vi "Combined Sim SubVI for 6.0.vi"(2 "Pressure Controls":T1, 3 "Line Flowrate Control":T1, 4 "Temperatures Control":T1) -> (0 "Flow Data":T3(array[cluster]), 1 "Rig Temperatures":T2)   [LabVIEW 2018]
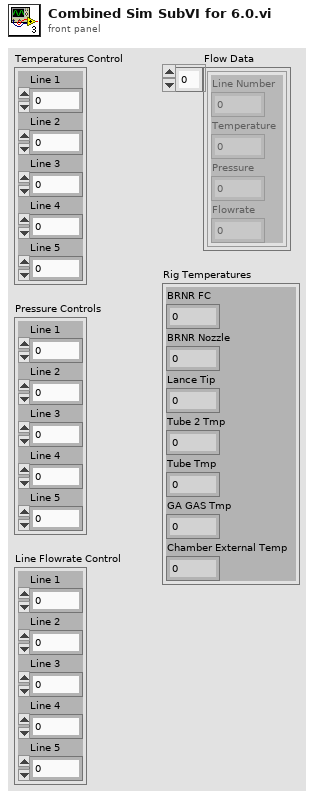
[diagram p1: front panel]
types:
  T1 = cluster{"Line 1":dbl, "Line 2":dbl, "Line 3":dbl, "Line 4":dbl, "Line 5":dbl}
  T2 = cluster{"BRNR FC":dbl, "BRNR Nozzle":dbl, "Lance Tip":dbl, "Tube 2 Tmp":dbl, "Tube Tmp":dbl, "GA GAS Tmp":dbl, "Chamber External Temp":dbl}
  T3 = cluster{"Line Number":dbl, "Temperature":dbl, "Pressure":dbl, "Flowrate":dbl}[]
  T4 = cluster{"Line Number":dbl, "Temperature":dbl, "Pressure":dbl, "Flowrate":dbl}
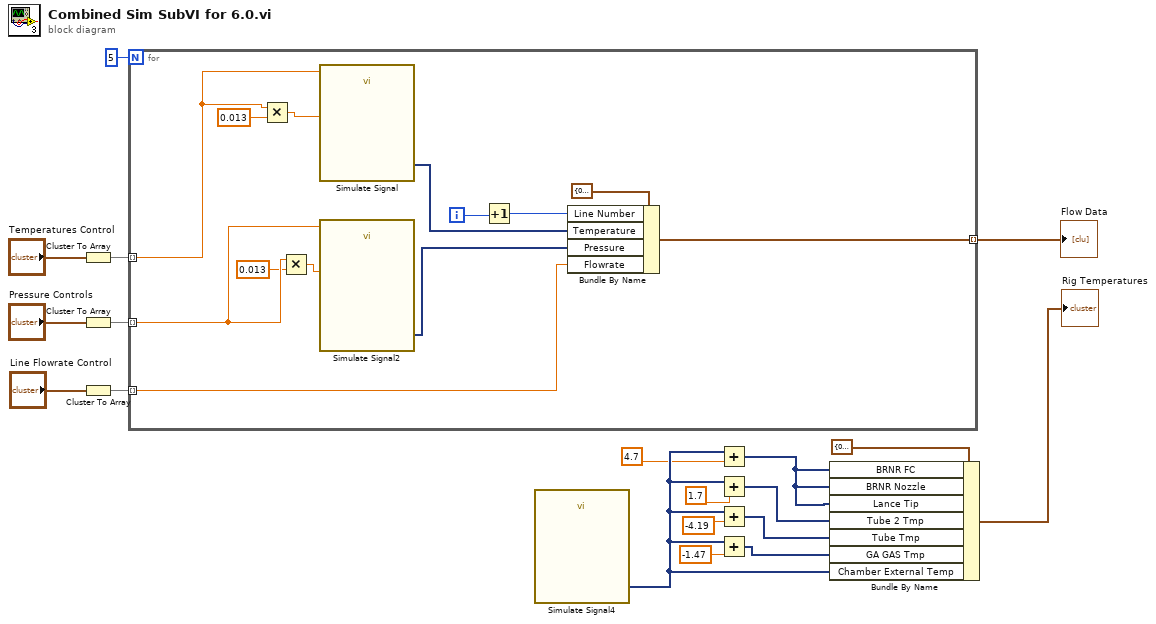
[diagram p0: block diagram]
diagram:
  n1 = Cluster To Array(cluster="Temperatures Control") -> (array=w12:dbl[])
  n2 = Cluster To Array(cluster="Pressure Controls") -> (array=w13:dbl[])
  n3 = Cluster To Array(cluster="Line Flowrate Control") -> (array=w14:dbl[])
  n4 = for {
    N: 5 -> [_]
    tunnel: [w32] -> w19 mode=indexing
    tunnel: w14 -> [w26] mode=indexing
    tunnel: w12 -> [w20] mode=indexing
    tunnel: w13 -> [w25] mode=indexing
    i -> [w30]
    n5 = Multiply(x=w20, y=0.013) -> (x*y=w21:dbl)
    n6 = Multiply(x=w25, y=0.013) -> (x*y=w23:dbl)
    n7 = call "Simulate Signal"("Offset"=w20, "Standard deviation"=w21) -> ("Temperature"=w29:dynamicdata)  [unwired: 12 in, 1 out]
    n8 = call "Simulate Signal2"("Offset"=w25, "Standard deviation"=w23) -> ("Pressure"=w27:dynamicdata)  [unwired: 12 in, 1 out]
    n9 = Increment(x=w30) -> (x+1=w28:i32)
    n10 = Bundle By Name(cluster=T4 {"Line Number"=0.0, "Temperature"=0.0, "Pressure"=0.0, "Flowrate"=0.0}, "Line Number"=w28, "Temperature"=w29, "Pressure"=w27, "Flowrate"=w26) -> (w32:T4)
  }
  "Flow Data" <- w19
  n11 = call "Simulate Signal4"() -> ("Rig Temperatures"=w10:dynamicdata)  [unwired: 14 in, 1 out]
  n12 = Add(x=w10, y=4.7) -> (x+y=w2:dynamicdata)
  n13 = Add(x=w10, y=1.7) -> (x+y=w4:dynamicdata)
  n14 = Add(x=w10, y=-4.19) -> (x+y=w6:dynamicdata)
  n15 = Add(x=w10, y=-1.47) -> (x+y=w8:dynamicdata)
  n16 = Bundle By Name(cluster=T2 {"BRNR FC"=0.0, "BRNR Nozzle"=0.0, "Lance Tip"=0.0, "Tube 2 Tmp"=0.0, "Tube Tmp"=0.0, "GA GAS Tmp"=0.0, "Chamber External Temp"=0.0}, "BRNR FC"=w2, "BRNR Nozzle"=w2, "Lance Tip"=w2, "Tube 2 Tmp"=w4, "Tube Tmp"=w6, "GA GAS Tmp"=w8, "Chamber External Temp"=w10) -> (→"Rig Temperatures":T2)
